vi "Logging Build Path.vi"(1 "number":i32, 2 "name":string="log", 3 "base path":path=path "c:/logs") -> (0 "built path":path)   [LabVIEW 2012, in "femtoRoboLib.lvlib"]
uses:
  femtoRoboLib.lvlib
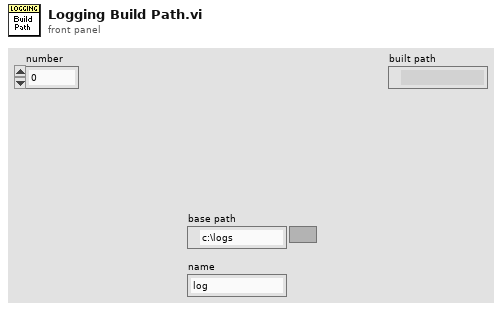
[diagram p1: front panel]
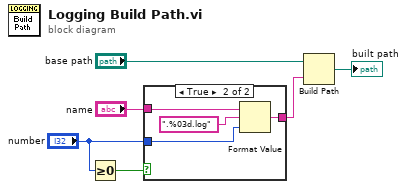
[diagram p0: block diagram]
diagram:
  n1 = Greater Or Equal To 0?(x="number") -> (x >= 0?=w2:bool)
  n2 = case shown="True" w2 {
    tunnel: [w7 w10] -> w6
    tunnel: "name" -> [w7 w9]
    tunnel: "number" -> [_ w8]
    frame False {
    }
    frame True {
      n3 = Format Value(string ("")=w9, format string=".%03d.log", value (0)=w8) -> (output string=w10:string)
    }
  }
  n4 = Build Path(base path="base path", name or relative path=w6) -> (appended path=→"built path":path)
